vi "Find_File.vi"() -> ()   [LabVIEW 2010]
panel:
  out "No of Hits":i32
  in  "Folder Path":path
  out "Files Found":path[](array[path])
  in  "Search Characters":string
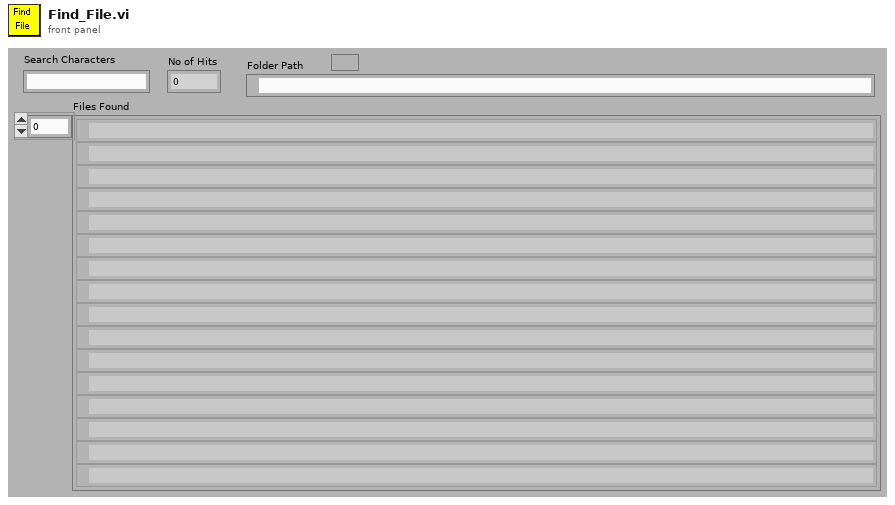
[diagram p1: front panel]
types:
  T1 = enum32{"existing file", "new file", "new or existing file", "existing dir", "new dir", "new or existing dir", "existing file (use LLBs)", "new file (use LLBs)", "new or existing file (use LLBs)", "new or existing file or directory (use LLBs)"}
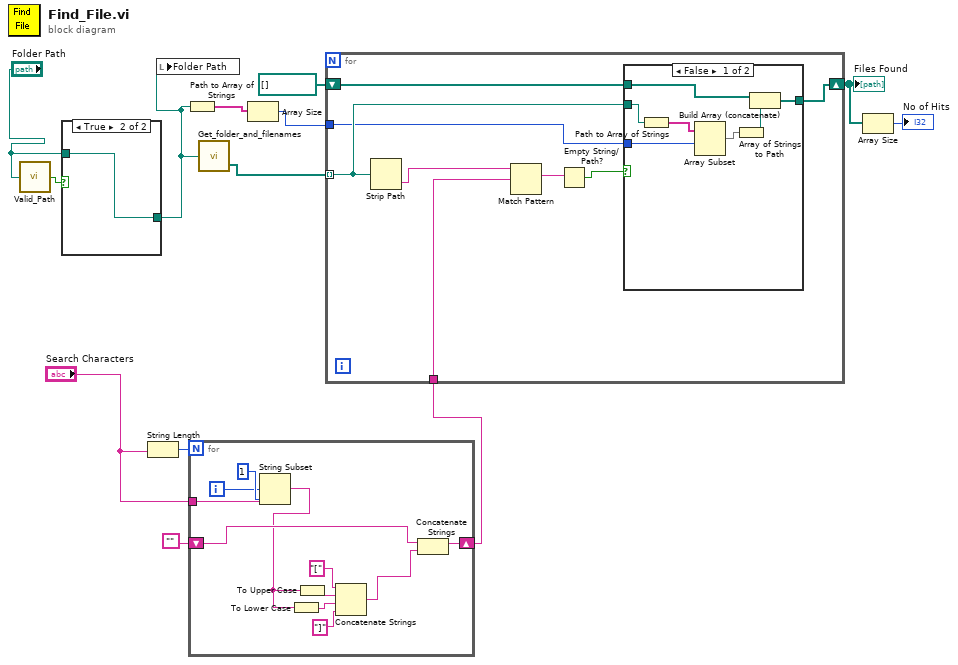
[diagram p0: block diagram]
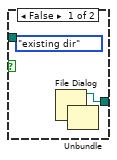
[diagram p2: hidden frame]
diagram:
  n1 = call "Valid_Path.vi"("Filename"="Folder Path") -> ("Valid Path?"=w3:bool)
  n2 = case shown="True" w3 {
    tunnel: [w15 w16] -> w2
    tunnel: "Folder Path" -> [_ w16]
    frame False {
      (unwired) T1."existing dir" ("select mode (2)")
      n3 = File Dialog() -> (0:w14:errorcluster, 3:w15:path)  [unwired: 1 in, 8 out]
      n4 = Unbundle(w14) -> ()  [unwired: 3 out]
    }
    frame True {
    }
  }
  n5 = String Length(string="Search Characters") -> (length=w13:i32)
  n6 = local write "Folder Path"(w2) -> ()
  n7 = Path to Array of Strings(0:w2) -> (2:w7:string[])  [unwired: 1 out]
  n8 = for {
    N: w13 -> [_]
    tunnel: "Search Characters" -> [w25]
    shift-right: [w23] -> w9
    shift-left: "" -> [w24]
    i -> [w26]
    n9 = String Subset(string=w25, offset (0)=w26, length (rest)=1 ("length")) -> (substring=w17:string)
    n10 = To Lower Case(string=w17) -> (all lower case string=w20:string)
    n11 = To Upper Case(1:w17) -> (0:w21:string)
    n12 = Concatenate Strings("[", w21, w20, "]" ("Substring")) -> (w22:string)
    n13 = Concatenate Strings(w24, w22) -> (w23:string)
  }
  n14 = call "Get_folder_and_filenames.vi"("file path (dialog if empty)"=w2) -> ("Files"=w10:path[])  [unwired: 1 out]
  n15 = Array Size(array=w7) -> (size(s)=w6:i32)
  n16 = for {
    tunnel: w10 -> [w30] mode=indexing
    shift-right: [w29] -> w5
    shift-left: path[] [] -> [w31]
    tunnel: w9 -> [w34]
    tunnel: w6 -> [w28]
    n17 = Strip Path(path=w30) -> (name=w35:string)  [unwired: 1 out]
    n18 = Match Pattern(string=w35, regular expression=w34) -> (match substring=w33:string)  [unwired: 4 out]
    n19 = Empty String/Path?(string/path=w33) -> (empty?=w32:bool)
    n20 = case shown="False" w32 {
      tunnel: w31 -> [w42 w43]
      tunnel: w30 -> [w39 _]
      tunnel: [w41 w43] -> w29
      tunnel: w28 -> [w36 _]
      frame False {
        n21 = Path to Array of Strings(0:w39) -> (2:w40:string[])  [unwired: 1 out]
        n22 = Array Subset(array=w40, index=w36) -> (w37:string[])  [unwired: 1 in]
        n23 = Array of Strings to Path(0:w37) -> (2:w38:path)  [unwired: 1 out]
        n24 = Build Array (concatenate)(w42, w38) -> (w41:path[])
      }
      frame True {
      }
    }
  }
  "Files Found" <- w5
  n25 = Array Size(array=w5) -> (size(s)=→"No of Hits":i32)
